vi "pointinirons.vi"(8 "Irons Range":dbl=45.0, 9 "Absolute Wind Direction":dbl, 10 "Boat location":T1 {"North" format="%#_10f"; "East" format="%#_8f"}, 11 "PointA":T1 {"North" format="%#_10f"; "East" format="%#_8f"}) -> (3 "In irons?":bool)   [LabVIEW 2013]
doc: "Checks if next waypoint will require sailing upwind into irons."
uses:
  Data/TypeDefs/UTM Location.ctl
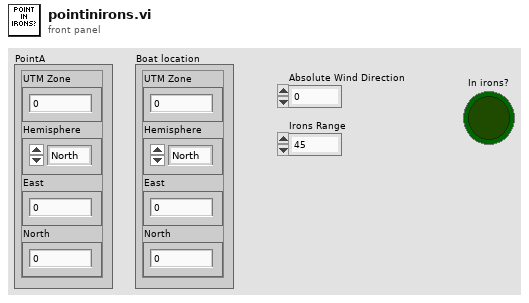
[diagram p1: front panel]
types:
  T1 = typedef "UTM Location.ctl" = cluster{"UTM Zone":dbl, "Hemisphere":enum16{"North", "South"}, "East":dbl, "North":dbl}
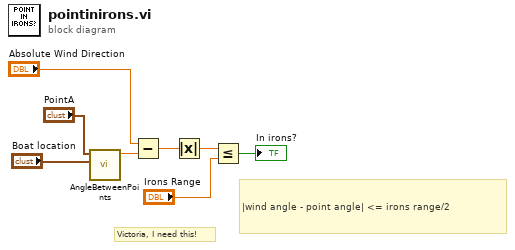
[diagram p0: block diagram]
diagram:
  # "|wind angle - point angle| <= irons range/2"
  # "Victoria, I need this!"
  n1 = call "AngleBetweenPoints.vi"("Point 2"="Boat location", "Point 1"="PointA") -> ("Angle from P1 to P2"=w1:dbl)  [unwired: 9 in]
  n2 = Subtract(x="Absolute Wind Direction", y=w1) -> (x-y=w6:dbl)
  n3 = Absolute Value(x=w6) -> (abs(x)=w5:dbl)
  n4 = Less Or Equal?(x=w5, y="Irons Range") -> (x <= y?=→"In irons?":bool)
